vi "Scan action.vi"(8 "error in (no error)":errorcluster, 11 "SweepControl in":refnum<class "Sweep Control.lvclass">) -> (0 "error out":errorcluster, 1 "Stop?":bool, 3 "SweepControl out":refnum<class "Sweep Control.lvclass">)   [LabVIEW 2019, in "Sweep Control.lvclass"]
uses:
  Sweep Control.lvclass
  Sweep Control.lvclass/Sweep Control.ctl
  <userlib>/LevyLab/Transport/Transport/Transport.lvclass/Transport.ctl
  <userlib>/LevyLab/Instrument Framework/Instrument Types/Cryostat/Typedefs/Magnet Mode--Enum.ctl
  <userlib>/LevyLab/Transport/Control Experiment/Control Experiment.lvclass/Control Experiment.ctl
  <userlib>/LevyLab/Transport/Transport/Transport.lvclass
  <userlib>/LevyLab/Transport/Control Experiment/Control Experiment.lvclass
  <userlib>/LevyLab/Instrument Framework/Instrument Types/Cryostat/Instrument.Cryostat.lvclass
  <userlib>/LevyLab/Instrument Framework/Instrument Types/Strain/Instrument.Strain.lvclass
  <userlib>/LevyLab/Instrument Framework/Instrument Types/Delay Line/Instrument.DelayLine.lvclass
  <userlib>/LevyLab/Lockin-Multichannel/Instrument.Lockin/Instrument.Lockin.lvclass
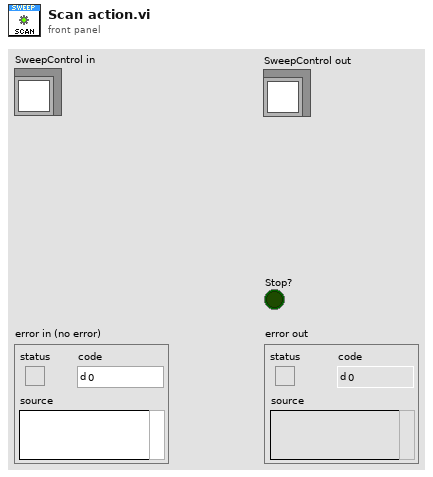
[diagram p1: front panel]
types:
  T1 = typedef "Sweep Control.lvclass/Cluster - Sweep Control.ctl" = cluster{"Start":dbl, "End":dbl, "Step":dbl, "Rate":dbl, "wait (ms/mK)":u32, "Address":string, "Priority":T2, "Scan name":T3, "Post Actions":T4[], "channel":i32}
  T2 = typedef "Sweep Control.lvclass/Enum - Priority.ctl" = enum16{"Priority 0", "Priority 1", "Priority 2", "Priority 3", "Priority 4", "Priority 5"}
  T3 = typedef "Sweep Control.lvclass/Enum - Action.ctl" = enum16{"OFF", "time", "Lockin Amplitude", "Lockin Frequency", "Lockin Bias", "Delay", "Strain", "DAQ Bias", "Magnet Field", "Temperature", "MW f1", "MW f2", "MW Amplitude1", "MW Amplitude2"}
  T4 = typedef "Sweep Control.lvclass/Enum - PostAction.ctl" = enum16{"Do Nothing", "Wait (time)", "Wait (Temperature)", "Wait (<T ; B sweep)", "Wait (Magnet)"}
  T5 = typedef "Sweep Control.lvclass/ScanParamters.ctl" = T6[]
  T6 = typedef "Sweep Control.lvclass/Cluster - ScanParamters.ctl" = cluster{"Start":dbl, "End":dbl, "Step":dbl, "Rate":dbl, "Waveform type":enum16{"linear", "triangle", "power"}, "wait (ms or K)":dbl, "Address":string, "channel":i32}
  T7 = typedef "Sweep Control.lvclass/ScanControl.ctl" = T8[]
  T8 = typedef "Sweep Control.lvclass/Cluster - ScanControl.ctl" = cluster{"Priority":T2, "Scan name":T3}
  T9 = typedef "Control Experiment.lvclass/Instrument Classes--cluster.ctl" = cluster{"KH7008":refnum<class "Instrument.KH7008.lvclass">[], "Lockin":refnum<class "Instrument.Lockin.lvclass">, "Temperature":refnum<class "Instrument.Cryostat.lvclass">, "Magnet":refnum<class "Instrument.Cryostat.lvclass">, "Rotator":refnum<class "Instrument.Cryostat.lvclass">, "Level":refnum<class "Instrument.Cryostat.lvclass">, "Capacitance Bridge":refnum<class "Instrument.CBridge.lvclass">, "Delay Line":refnum<class "Instrument.DelayLine.lvclass">, "Strain Cell":refnum<class "Instrument.Strain.lvclass">, "VNA":refnum<class "Instrument.VNA.lvclass">, "Voltage Source":refnum<class "Instrument.VSource.lvclass">}
  T10 = typedef "Instrument.Cryostat.lvclass/Magnet Mode--Enum.ctl" = enum16{"Persistent", "Driven"}
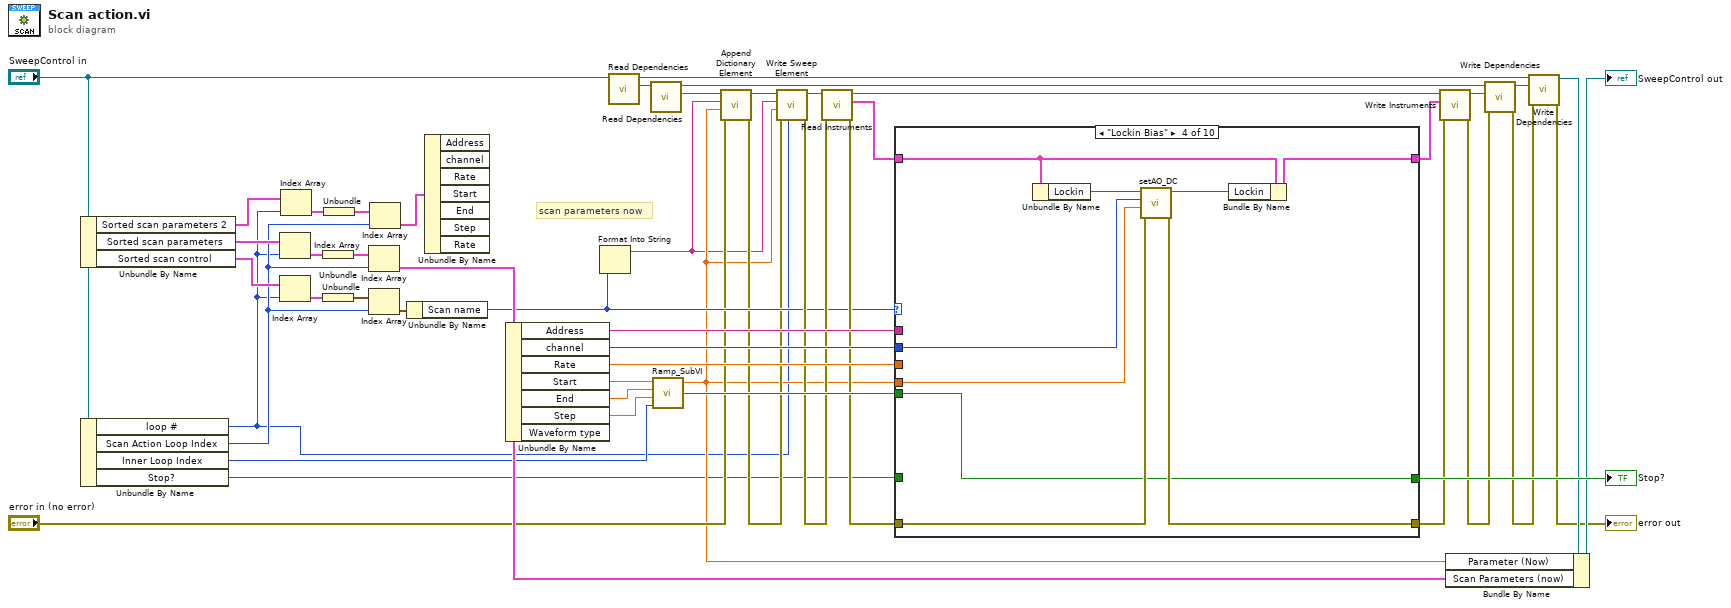
[diagram p0: block diagram]
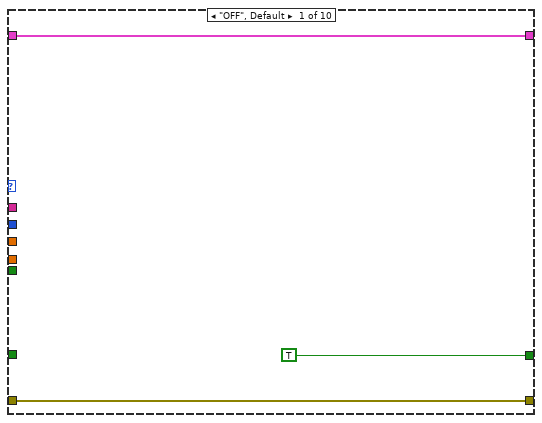
[diagram p2: hidden frame]
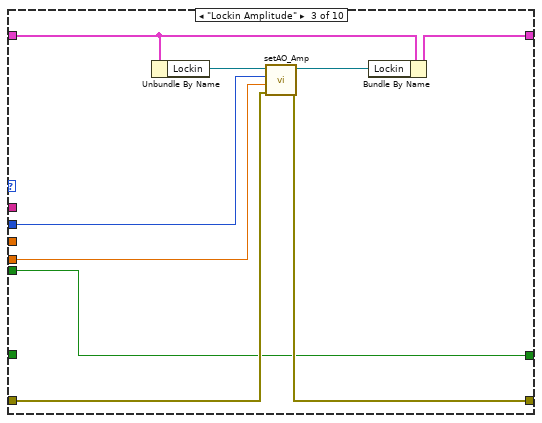
[diagram p4: hidden frame]
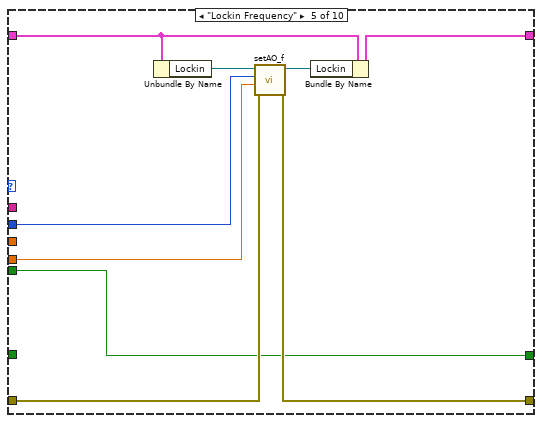
[diagram p5: hidden frame]
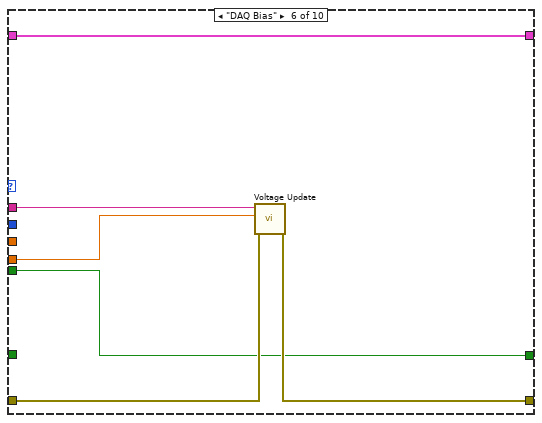
[diagram p6: hidden frame]
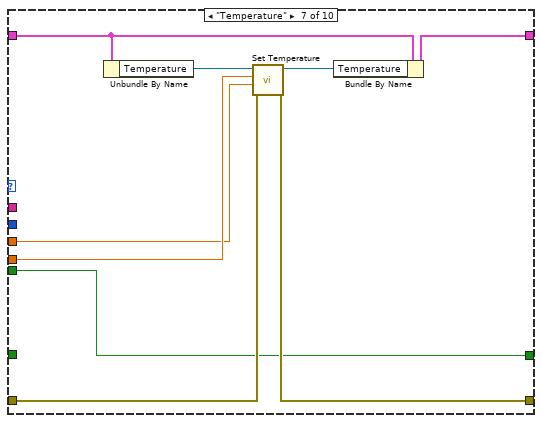
[diagram p7: hidden frame]
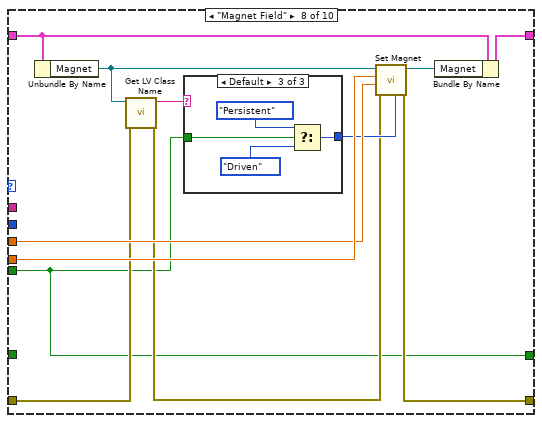
[diagram p8: hidden frame]
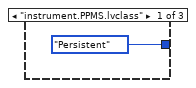
[diagram p9: hidden frame]
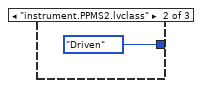
[diagram p10: hidden frame]
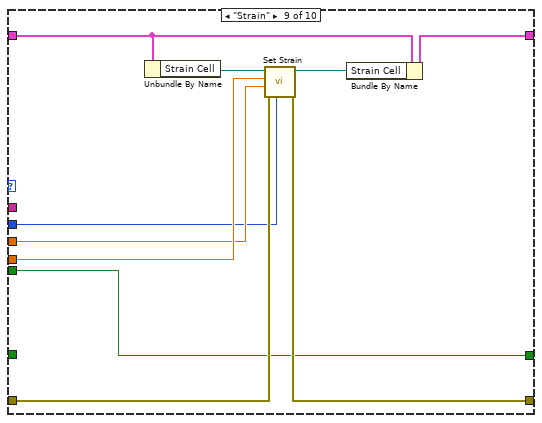
[diagram p11: hidden frame]
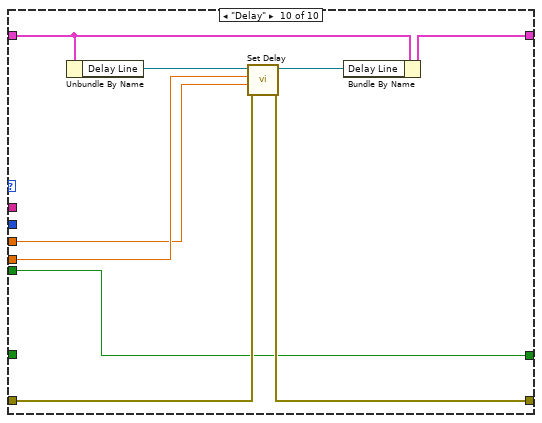
[diagram p12: hidden frame]
diagram:
  # "scan parameters now"
  n1 = Unbundle By Name("SweepControl in") -> ("Sorted scan parameters 2"=w3:cluster{"Scan parameters 2":T1[]}[], "Sorted scan parameters"=w42:cluster{T5}[], "Sorted scan control"=w36:cluster{T7}[])
  n2 = Unbundle By Name("SweepControl in") -> ("loop #"=w9:i32, "Scan Action Loop Index"=w15:i32, "Inner Loop Index"=w19:i32, "Stop?"=w18:bool)
  n3 = Index Array(array=w42, index=w9) -> (element=w41:cluster{T5})
  n4 = Index Array(array=w36, index=w9) -> (element=w38:cluster{T7})
  n5 = Index Array(array=w3, index=w9) -> (element=w16:cluster{"Scan parameters 2":T1[]})
  n6 = Unbundle(w41) -> (w40:T5)
  n7 = Unbundle(w38) -> (w39:T7)
  n8 = Unbundle(w16) -> ("Scan parameters 2"=w17:T1[])
  n9 = Index Array(array=w40, index=w15) -> (element=w29:T6)
  n10 = Index Array(array=w39, index=w15) -> (element=w37:T8)
  n11 = Index Array(array=w17, index=w15) -> (element=w14:T1)
  n12 = Unbundle By Name(w37) -> ("Scan name"=w28:T3)
  n13 = Unbundle By Name(w14) -> ()  [unwired: 7 out]
  n14 = Unbundle By Name(w29) -> ("Address"=w47:string, "channel"=w49:i32, "Rate"=w44:dbl, "Start"=w46:dbl, "End"=w35:dbl, "Step"=w34:dbl)  [unwired: 1 out]
  n15 = Format Into String(w28) -> (resulting string=w23:string)  [unwired: 3 in, 1 out]
  n16 = call <userlib>:"Read Dependencies.vi"("SweepControl in"="SweepControl in") -> ("Transport"=w5:refnum<class "Transport.lvclass">, "SweepControl out"=w4:refnum<class "Sweep Control.lvclass">)  [unwired: 8 in, 1 out]
  n17 = call <userlib>:"Read Dependencies.vi"("Transport"=w5) -> ("C.E."=w13:refnum<class "Control Experiment.lvclass">, "Transport"=w11:refnum<class "Transport.lvclass">)  [unwired: 8 in, 1 out]
  n18 = call <userlib>:"Ramp_SubVI.vi"("index"=w19, "step"=w34, "end"=w35, "start"=w46) -> ("Stop?"=w45:bool, "Numeric"=w24:dbl)  [unwired: 1 in]
  n19 = call <userlib>:"Append Dictionary Element.vi"("error in (no error)"="error in (no error)", "value"=w24, "key"=w23, "Control Experiment in"=w13) -> ("error out"=w26:errorcluster, "Control Experiment out"=w25:refnum<class "Control Experiment.lvclass">)  [unwired: 6 in]
  n20 = call <userlib>:"Write Sweep Element.vi"("loop index"=w9, "error in (no error)"=w26, "value"=w24, "key"=w23, "Control Experiment in"=w25) -> ("error out"=w32:errorcluster, "Control Experiment out"=w33:refnum<class "Control Experiment.lvclass">)  [unwired: 5 in]
  n21 = call <userlib>:"Read Instruments.vi"("error in (no error)"=w32, "Control Experiment in"=w33) -> ("error out"=w31:errorcluster, "Instruments"=w30:T9, "Control Experiment out"=w22:refnum<class "Control Experiment.lvclass">)  [unwired: 7 in]
  n22 = case shown="\"Lockin Bias\"" w28 {
    tunnel: w49 -> [_ _ w62 w73 w82 _ _ _ w120 _]
    tunnel: [TRUE ("Stop?") w55 w56 w65 w74 w84 w89 w98 w116 w126] -> w48
    tunnel: w47 -> [_ _ _ _ _ w86 _ _ _ _]
    tunnel: w24 -> [_ _ w61 w72 w81 w83 w97 w108 w124 w131]
    tunnel: w45 -> [_ _ w56 w65 w74 w84 w89 w98 w116 w126]
    tunnel: w44 -> [_ _ _ _ _ _ w93 w107 w123 w130]
    tunnel: [w51 w54 w60 w71 w80 w88 w96 w109 w121 w132] -> w21
    tunnel: w30 -> [w50 w53 w58 w68 w75 w85 w91 w101 w118 w128]
    tunnel: w31 -> [w51 w54 w64 w69 w78 w87 w94 w103 w122 w133]
    tunnel: w18 -> [_ w55 _ _ _ _ _ _ _ _]
    tunnel: [w50 w53 w57 w66 w76 w85 w90 w99 w117 w127] -> w20
    frame "OFF", Default {
    }
    frame "time" {
    }
    frame "Lockin Amplitude" {
      n23 = Unbundle By Name(w58) -> ("Lockin"=w63:refnum<class "Instrument.Lockin.lvclass">)
      n24 = call <userlib>:"setAO_Amp.vi"("error in (no error)"=w64, "Amplitude (V)"=w61, "AO Channel"=w62, "Instrument.Lockin in"=w63) -> ("error out"=w60:errorcluster, "Instrument.Lockin out"=w59:refnum<class "Instrument.Lockin.lvclass">)  [unwired: 6 in]
      n25 = Bundle By Name(cluster=w58, "Lockin"=w59) -> (w57:T9)
    }
    frame "Lockin Bias" {
      n26 = Unbundle By Name(w68) -> ("Lockin"=w70:refnum<class "Instrument.Lockin.lvclass">)
      n27 = call <userlib>:"setAO_DC.vi"("error in (no error)"=w69, "DC (V)"=w72, "AO Channel"=w73, "Instrument.Lockin in"=w70) -> ("error out"=w71:errorcluster, "Instrument.Lockin out"=w67:refnum<class "Instrument.Lockin.lvclass">)  [unwired: 6 in]
      n28 = Bundle By Name(cluster=w68, "Lockin"=w67) -> (w66:T9)
    }
    frame "Lockin Frequency" {
      n29 = Unbundle By Name(w75) -> ("Lockin"=w79:refnum<class "Instrument.Lockin.lvclass">)
      n30 = call <userlib>:"setAO_f.vi"("error in (no error)"=w78, "Frequency (Hz)"=w81, "AO Channel"=w82, "Instrument.Lockin in"=w79) -> ("error out"=w80:errorcluster, "Instrument.Lockin out"=w77:refnum<class "Instrument.Lockin.lvclass">)  [unwired: 6 in]
      n31 = Bundle By Name(cluster=w75, "Lockin"=w77) -> (w76:T9)
    }
    frame "DAQ Bias" {
      n32 = call <userlib>:"Voltage Update.vi"("error in (no error)"=w87, "Voltage Output"=w83, "Physical Channel"=w86) -> ("error out"=w88:errorcluster)  [unwired: 6 in, 2 out]
    }
    frame "Temperature" {
      n33 = Unbundle By Name(w91) -> ("Temperature"=w95:refnum<class "Instrument.Cryostat.lvclass">)
      n34 = call-dynamic "Set Temperature.vi"("error in (no error)"=w94, "Rate (K/min)"=w93, "Temperature (K)"=w97, "Instrument.Cryostat in"=w95) -> ("error out"=w96:errorcluster, "Instrument.Cryostat out"=w92:refnum<class "Instrument.Cryostat.lvclass">)  [unwired: 6 in]
      n35 = Bundle By Name(cluster=w91, "Temperature"=w92) -> (w90:T9)
    }
    frame "Magnet Field" {
      n36 = Unbundle By Name(w101) -> ("Magnet"=w105:refnum<class "Instrument.Cryostat.lvclass">)
      n37 = call <vilib>:"Get LV Class Name.vi"("error in (no error)"=w103, "object"=w105) -> ("error out"=w102:errorcluster, "class name"=w104:string)  [unwired: 8 in]
      n38 = case shown="Default" w104 {
        tunnel: w98 -> [_ _ w112]
        tunnel: [Magnet_Mode--Enum."Persistent" ("Mode") Magnet_Mode--Enum."Driven" ("Mode") w115] -> w106
        frame "instrument.PPMS.lvclass" {
        }
        frame "instrument.PPMS2.lvclass" {
        }
        frame Default {
          n39 = Select(t=Magnet_Mode--Enum."Persistent" ("Mode"), s=w112, f=Magnet_Mode--Enum."Driven" ("Mode")) -> (s? t:f=w115:T10)
        }
      }
      n40 = call-dynamic "Set Magnet.vi"("Mode"=w106, "error in (no error)"=w102, "Target Rate (T/min)"=w107, "Target Field (T)"=w108, "Instrument.Cryostat in"=w105) -> ("error out"=w109:errorcluster, "Instrument.Cryostat out"=w100:refnum<class "Instrument.Cryostat.lvclass">)  [unwired: 5 in]
      n41 = Bundle By Name(cluster=w101, "Magnet"=w100) -> (w99:T9)
    }
    frame "Strain" {
      n42 = Unbundle By Name(w118) -> ("Strain Cell"=w125:refnum<class "Instrument.Strain.lvclass">)
      n43 = call-dynamic "Set Strain.vi"("Channel"=w120, "error in (no error)"=w122, "Slew (V/s)"=w123, "Strain (V)"=w124, "Instrument.Strain in"=w125) -> ("error out"=w121:errorcluster, "Instrument.Strain out"=w119:refnum<class "Instrument.Strain.lvclass">)  [unwired: 5 in]
      n44 = Bundle By Name(cluster=w118, "Strain Cell"=w119) -> (w117:T9)
    }
    frame "Delay" {
      n45 = Unbundle By Name(w128) -> ("Delay Line"=w134:refnum<class "Instrument.DelayLine.lvclass">)
      n46 = call-dynamic "Set Delay.vi"("error in (no error)"=w133, "Rate (ps/s)"=w130, "Delay (ps)"=w131, "Instrument.Delay in"=w134) -> ("error out"=w132:errorcluster, "Instrument.Delay out"=w129:refnum<class "Instrument.DelayLine.lvclass">)  [unwired: 6 in]
      n47 = Bundle By Name(cluster=w128, "Delay Line"=w129) -> (w127:T9)
    }
  }
  "Stop?" <- w48
  n48 = call <userlib>:"Write Instruments.vi"("error in (no error)"=w21, "Instruments"=w20, "Control Experiment in"=w22) -> ("error out"=w10:errorcluster, "Control Experiment out"=w12:refnum<class "Control Experiment.lvclass">)  [unwired: 7 in]
  n49 = call <userlib>:"Write Dependencies.vi"("error in (no error)"=w10, "Control Experiment"=w12, "Transport in"=w11) -> ("error out"=w2:errorcluster, "Transport out"=w8:refnum<class "Transport.lvclass">)  [unwired: 7 in]
  n50 = call <userlib>:"Write Dependencies.vi"("error in (no error)"=w2, "Transport"=w8, "SweepControl in"=w4) -> ("error out"=→"error out":errorcluster, "SweepControl out"=w7:refnum<class "Sweep Control.lvclass">)  [unwired: 7 in]
  n51 = Bundle By Name(cluster=w7, "Parameter (Now)"=w24, "Scan Parameters (now)"=w29) -> (→"SweepControl out":refnum<class "Sweep Control.lvclass">)
